vi "线灰度曲线设置.vi"(8 "error in (no error)":errorcluster, 11 "Image Src":T1) -> (0 "error out":errorcluster, 1 "关闭":bool, 2 "分析图":cluster{"x0":sgl, "dx":sgl, "Pixels Line":sgl[]}(graph), 3 "图像":T1(plugin-control))   [LabVIEW 2018]
uses:
  <vilib>/vision/Image Controls.llb/IMAQ Image.ctl
  <vilib>/vision/NI_Vision_Development_Module.lvlib
panel:
  in  "关闭":bool
  in  "颜色":u32(colorbox)=16711680
  in  "终点":cluster{"X":i32, "Y":i32}={"X"=0, "Y"=180}
  in  "起点":cluster{"X":i32, "Y":i32}={"X"=0, "Y"=180}
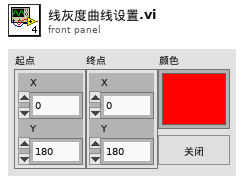
[diagram p1: front panel]
types:
  T1 = typedef "IMAQ Image.ctl" = refnum<image>
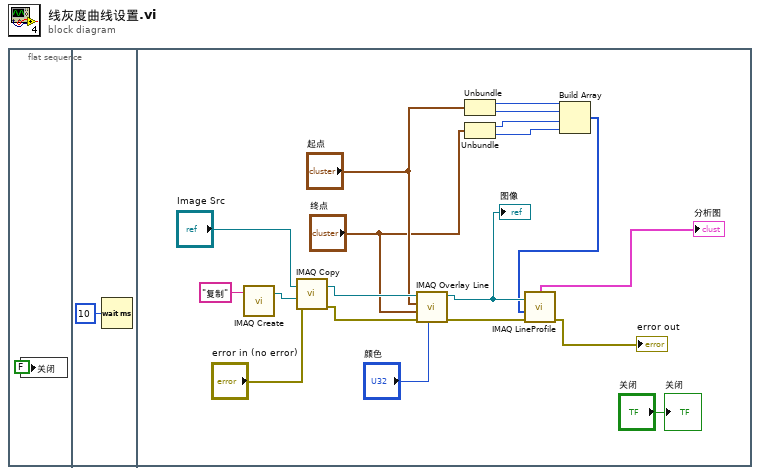
[diagram p0: block diagram]
diagram:
  n1 = flat-sequence {
    frame #0 {
      n2 = local write "关闭"(FALSE ("关闭")) -> ()
    }
    frame #1 {
      n3 = Wait (ms)(milliseconds to wait=u32 10 ("等待时间（毫秒）")) -> ()  [unwired: 1 out]
    }
    frame #2 {
      n4 = call "IMAQ Create"("Image Name"="复制") -> ("New Image"=w19:T1)  [unwired: 4 in, 1 out]
      n5 = call "IMAQ Copy"("error in (no error)"="error in (no error)", "Image Dst"=w19, "Image Src"="Image Src") -> ("error out"=w17:errorcluster, "Image Dst Out"=w18:T1)  [unwired: 3 in]
      n6 = call "IMAQ Overlay Line"("Color"="颜色", "error in (no error)"=w17, "End Point"="终点", "Start Point"="起点", "Image"=w18) -> ("error out"=w14:errorcluster, "Image Out"=w12:T1)  [unwired: 5 in]
      "图像" <- w12
      n7 = Unbundle("起点") -> ("X"=w9:i32, "Y"=w8:i32)
      n8 = Unbundle("终点") -> ("X"=w7:i32, "Y"=w6:i32)
      n9 = Build Array(w9, w8, w7, w6) -> (w5:i32[])
      n10 = call "IMAQ LineProfile"("error in (no error)"=w14, "Line Coordinates"=w5, "Image"=w12) -> ("error out"=→"error out":errorcluster, "Line Graph"=→"分析图":cluster{"x0":sgl, "dx":sgl, "Pixels Line":sgl[]})  [unwired: 2 in, 2 out]
      "关闭" <- "关闭"
    }
  }
